vi "KacperLabView1.vi"() -> ()   [LabVIEW 2014]
panel:
  in  "stop":bool
  in  "Knob 2":dbl(knob) scale=0.0..10.0
  in  "Knob":dbl(knob) scale=0.0..10.0
  out "Waveform Graph":dynamicdata(graph)
  out "Numeric":dbl
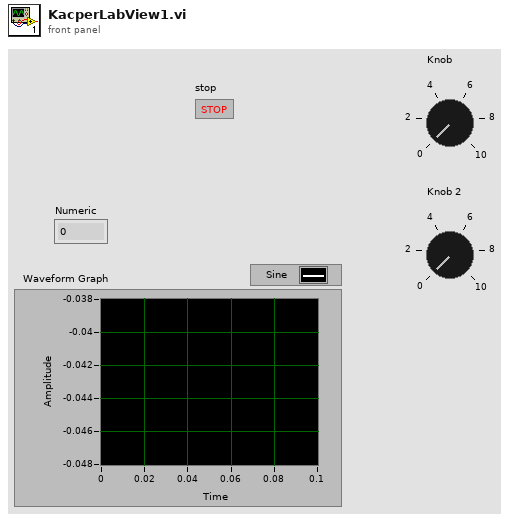
[diagram p1: front panel]
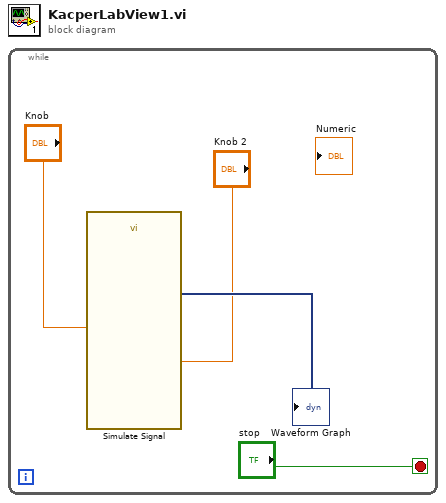
[diagram p0: block diagram]
diagram:
  n1 = while {
    stop <- "stop" stop-if-true
    n2 = call "Simulate Signal"("Frequency"="Knob 2", "Amplitude"="Knob") -> ("Sine"=→"Waveform Graph":dynamicdata)  [unwired: 12 in, 1 out]
  }
